vi "niRFUtil ERR Error In to Error Code.vi"(7 "error in (no error)":errorcluster) -> (8 "Error Code":T1)   [LabVIEW 2015, in "niRFUtil.lvlib"]
doc: "This utility is used to strip off the error code from a LabVIEW error cluster.\n\n(c) Copyright 2008, National Instruments, Inc. This software may not be duplicated, sold, or distributed without written consent from National Instruments."
uses:
  niRFUtil.lvlib
  Includes/niRFUtil INC Error Code.ctl
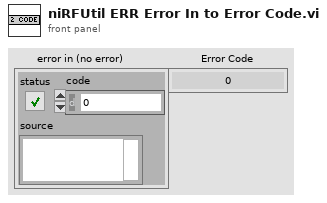
[diagram p1: front panel]
types:
  T1 = typedef "niRFUtil.lvlib/niRFUtil INC Error Code.ctl" = i32
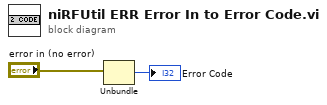
[diagram p0: block diagram]
diagram:
  n1 = Unbundle("error in (no error)") -> ("code"=→"Error Code":i32)  [unwired: 2 out]
